vi "Test VIP Uninstall Job.vi"() -> ()   [LabVIEW 2014]
uses:
  Core/LabVIEW CI Service/Extensions/VIP Uninstall/VIP Uninstall/VIP Uninstall - STYP.ctl
  Core/LabVIEW CI Service/Classes/Status Updater/Status Updater.lvclass/Status Updater.ctl
  Core/LabVIEW CI Service/Classes/Job/Job.lvclass/Job.ctl
  Core/LabVIEW CI Service/Extensions/VIP Uninstall/VIP Uninstall/VIP Uninstall.lvclass
  Core/LabVIEW CI Service/Classes/Status Updater/Status Updater.lvclass
  Core/LabVIEW CI Service/Classes/Job/Job.lvclass
panel:
  in  "VIP Name":string
  in  "LabVIEW Version":string="14.0"
  in  "Workspace Path":path=path "P:/alsmith/Sales/users/ACS/LabVIEW Continuous Integration/Jenkins Sample Project/Run VI Golden DUT.vi"
  out "Results":T1 {"Status" items=["Service Error"=504, "Abort"=503, "Fail"=500, "Pass"=200]}
  out "Steps":string[](array[string])
  out "Progress Percents":u32[](array[numeric])
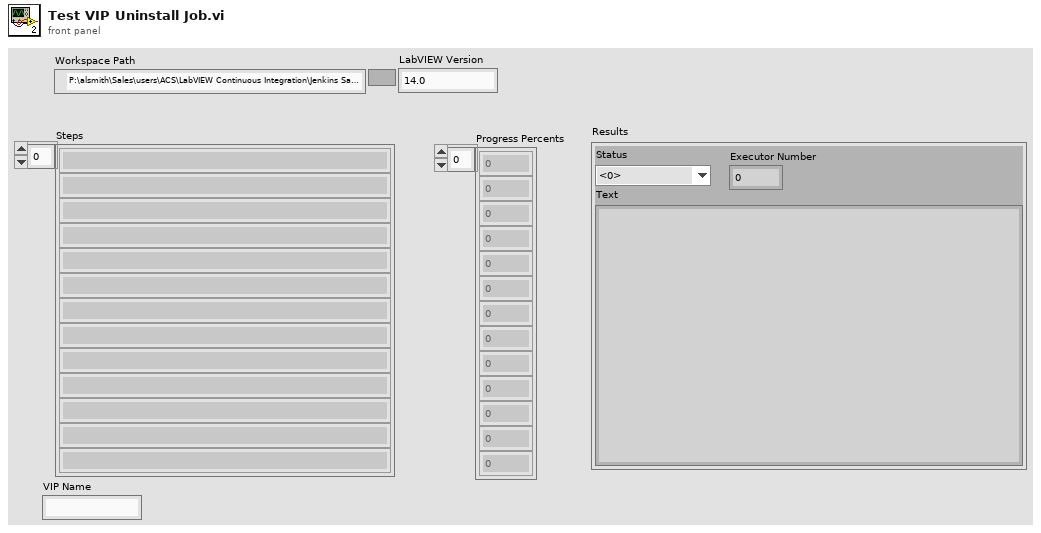
[diagram p1: front panel]
types:
  T1 = cluster{"Status":u16, "Text":string, "Executor Number":i32}
  T2 = typedef "VIP Uninstall - STYP.ctl" = cluster{"VIP Name":string, "LabVIEW Version":string}
  T3 = cluster{"Event Registration Refnum":refnum<event-registration>, "Event Registration Refnum":refnum<event-registration>}
  T4 = typedef "Job Results - STYP.ctl" = cluster{"Status":u16, "Text":string, "Executor Number":i32}
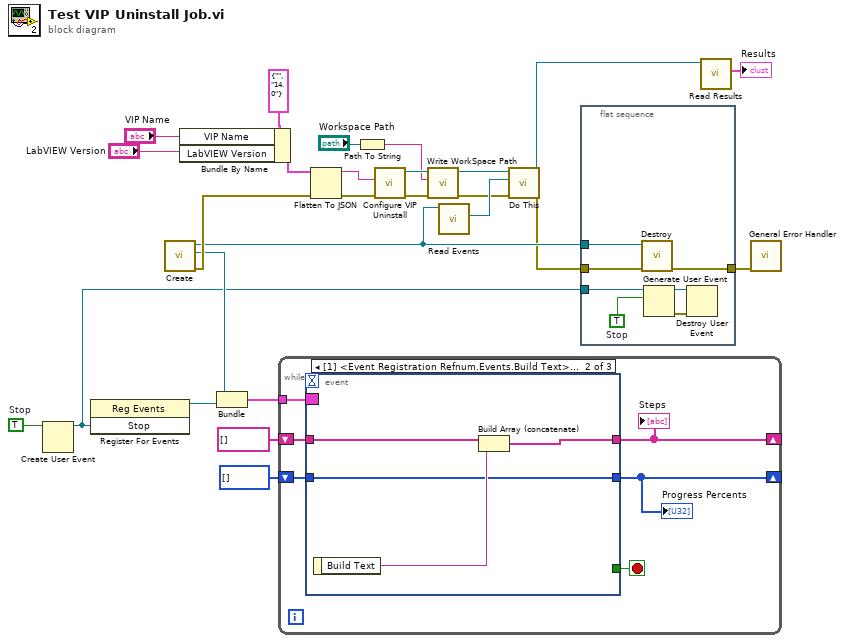
[diagram p0: block diagram]
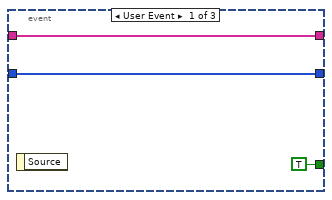
[diagram p2: hidden frame]
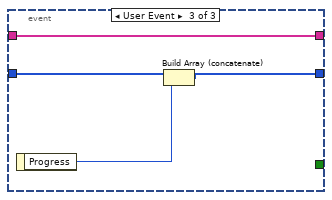
[diagram p3: hidden frame]
diagram:
  w24 = TRUE  # Stop
  n1 = Create User Event(user event datatype=w24) -> (user event=w20:refnum<user-event>)  [unwired: 1 in, 1 out]
  n2 = register-events(w20) -> (reference out=w21:refnum<event-registration>)  [unwired: 2 in, 1 out]
  n3 = call "Create.vi"() -> ("error out"=w25:errorcluster, "Event Registration Refnum"=w23:refnum<event-registration>, "Status Updater out"=w15:refnum<class "Status Updater.lvclass">)  [unwired: 9 in]
  n4 = Bundle By Name(cluster=T2 {"VIP Name"="", "LabVIEW Version"="14.0"} ("VIP Uninstall"), "VIP Name"="VIP Name", "LabVIEW Version"="LabVIEW Version") -> (w26:T2)
  n5 = Bundle("Event Registration Refnum"=w23, "Event Registration Refnum"=w21) -> (w22:T3)  [unwired: 1 in]
  n6 = while {
    tunnel: w22 -> [w32]
    shift-right: [w28] -> _
    shift-left: string[] [] -> [w30]
    shift-right: [w27] -> _
    shift-left: u32[] [] -> [w29]
    stop <- w31 stop-if-true
    n7 = event shown="[1] <Event Registration Refnum.Events.Build Text>: User Event" {
      selector: w32 -> [_ _ _]
      dyn-events: _ -> [_ _ _]
      timeout: _ -> [_ _ _]
      tunnel: [TRUE _ _] -> w31
      tunnel: w30 -> [w34 w39 w43]
      tunnel: [w34 w38 w43] -> w28
      tunnel: w29 -> [w33 w36 w42]
      tunnel: [w33 w36 w41] -> w27
      event User Event {
        n8 = event-data() -> ()  [unwired: 1 in, 1 out]
      }
      event User Event {
        n9 = event-data() -> ("Build Text"=w37:string)  [unwired: 1 in]
        n10 = Build Array (concatenate)(w39, w37) -> (w38:string[])
      }
      event User Event {
        n11 = event-data() -> ("Progress"=w40:u32)  [unwired: 1 in]
        n12 = Build Array (concatenate)(w42, w40) -> (w41:u32[])
      }
    }
    "Steps" <- w28
    "Progress Percents" <- w27
  }
  n13 = Flatten To JSON(anything=w26, error in (no error)=w25) -> (JSON string=w13:string, 11:w14:errorcluster)  [unwired: 1 in]
  n14 = Path To String(path="Workspace Path") -> (string=w5:string)
  n15 = call "Configure VIP Uninstall.vi"("error in (no error)"=w14, "JSON string"=w13) -> ("error out"=w6:errorcluster, "VIP Install Out"=w7:refnum<class "VIP Uninstall.lvclass">)  [unwired: 8 in]
  n16 = call "Write WorkSpace Path.vi"("error in (no error)"=w6, "WorkSpace Path"=w5, "Job in"=w7) -> ("error out"=w3:errorcluster, "Job out"=w4:refnum<class "VIP Uninstall.lvclass">)  [unwired: 7 in]
  n17 = call "Read Events.vi"("Status Updater in"=w15) -> ("Status Events"=w11:refnum<class "Status Events.lvclass">)  [unwired: 10 in]
  n18 = call-dynamic "Do This.vi"("error in (no error)"=w3, "Status Events"=w11, "VIP Uninstall in"=w4) -> ("error out"=w9:errorcluster, "VIP Uninstall out"=w10:refnum<class "VIP Uninstall.lvclass">)  [unwired: 7 in]
  n19 = flat-sequence {
    tunnel: w15 -> [w50]
    tunnel: w9 -> [w49]
    tunnel: w20 -> [w47]
    tunnel: [w46] -> w17
    frame #0 {
      w48 = TRUE  # Stop
      n20 = call "Destroy.vi"("error in (no error)"=w49, "Status Updater in"=w50) -> ("error out"=w46:errorcluster)  [unwired: 9 in]
      n21 = Generate User Event(user event=w47, event data cluster=w48) -> (user event out=w44:refnum<user-event>, error out=w45:errorcluster)  [unwired: 2 in]
      n22 = Destroy User Event(user event=w44, error in=w45) -> ()  [unwired: 1 out]
    }
  }
  n23 = call "Read Results.vi"("Job in"=w10) -> ("Results"=→"Results":T4)  [unwired: 10 in]
  n24 = call <vilib>:"General Error Handler.vi"("error in (no error)"=w17) -> ()  [unwired: 10 in, 5 out]
